vi "GPIO Write Direction.vi"(7 "GPIO #":T2=-1, 8 "error in (no error)":errorcluster, 10 "GPIO Direction":T1, 11 "FirmwareComms in":refnum<class "VisaComms.lvclass">) -> (0 "error out":errorcluster, 3 "FirmwareComms out":refnum<class "VisaComms.lvclass">)   [LabVIEW 2024, in "CTI.lvlib" / "VisaComms.lvclass"]
uses:
  VisaComms.lvclass
  GPIO Number.ctl
  GPIO Direction.ctl
  VisaComms.lvclass/VisaComms.ctl
  Clean Visa Errors.vi
  CTI.lvlib
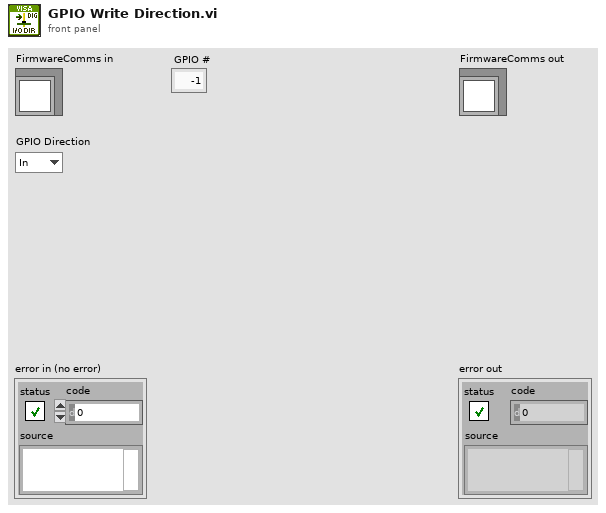
[diagram p1: front panel]
types:
  T1 = typedef "CTI.lvlib/GPIO Direction.ctl" = enum16{"In", "Out"}
  T2 = typedef "CTI.lvlib/GPIO Number.ctl" = i8
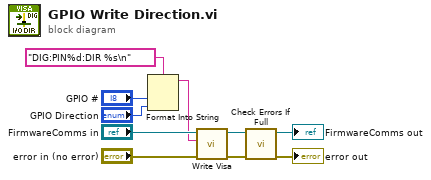
[diagram p0: block diagram]
diagram:
  n1 = Format Into String(format string="DIG:PIN%d:DIR %s\n", "GPIO #", "GPIO Direction") -> (resulting string=w4:string)  [unwired: 2 in, 1 out]
  n2 = call "Write Visa.vi"("error in (no error)"="error in (no error)", "write buffer"=w4, "VisaComms in"="FirmwareComms in") -> ("error out"=w2:errorcluster, "VisaComms out"=w6:refnum<class "VisaComms.lvclass">)  [unwired: 6 in, 1 out]
  n3 = call "Check Errors If Full.vi"("error in (no error)"=w2, "VisaComms in"=w6) -> ("error out"=→"error out":errorcluster, "VisaComms out"=→"FirmwareComms out":refnum<class "VisaComms.lvclass">)  [unwired: 8 in]
